vi "Increment Message Count.vi"(11 "Process In":refnum<class "Process.lvclass">) -> (3 "Process Out":refnum<class "Process.lvclass">)   [LabVIEW 2020, in "Process.lvclass"]
doc: "Clears the in process loop flag. This VI should be called if a branch of the process instance is sent out of the process loop to avoid undefined behavior."
uses:
  Process.lvclass
  Process.lvclass/Process.ctl
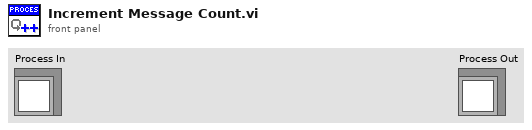
[diagram p1: front panel]
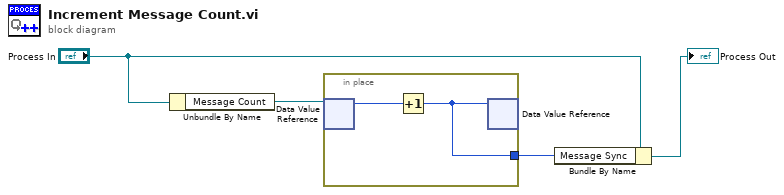
[diagram p0: block diagram]
diagram:
  n1 = Unbundle By Name("Process In") -> ("Message Count"=w4:refnum<data-value>)
  n2 = in-place {
    in-place-border: [w5] -> w1
    n3 = in-place-dvr #1(w4) -> (w6:u16)  [unwired: 1 out]
    n4 = Increment(x=w6) -> (x+1=w5:u16)
    n5 = in-place-dvr #1(w5) -> ()  [unwired: 2 out]
  }
  n6 = Bundle By Name(cluster="Process In", "Message Sync"=w1) -> (→"Process Out":refnum<class "Process.lvclass">)
